vi "phan.vi"() -> ()   [LabVIEW 2019]
uses:
  <vilib>/Platform/TimedLoop/XDataNode/timing_clust.ctl
  <vilib>/Platform/TimedLoop/XDataNode/nitl_modes.ctl
  <vilib>/Platform/TimedLoop/XDataNode/wakeup.ctl
  <vilib>/platform/TimedLoop/XDataNode/XDataNode.xnode
  <vilib>/Platform/TimedLoop/XDataNode/XDNodeRunTimeDep.lvlib
  <vilib>/ptbypt/NI_PtbyPt.lvlib
panel:
  in  "Kdv3":dbl
  in  "Kiv3":dbl=30.0
  in  "Kpv3":dbl=0.6
  in  "Kdv2":dbl
  in  "Kiv2":dbl=30.0
  in  "Kpv2":dbl=0.6
  in  "1000Ts":i64=200
  out "fs":dbl=10.0
  out "TOA DO 2":dbl[][](array[numeric])
  out "sailechS":cluster{"Filtered x":dbl}(graph)
  in  "Kds":dbl
  in  "Kis":dbl
  in  "Kps":dbl=4.0
  in  "?":enum32{"DUONG 2", "DUONGTRON"}(tab)
  in  "S_sp 2":dbl=0.13
  in  "R 2":dbl=0.5
  in  "phi_end 2":dbl=100.0
  in  "R":dbl=0.5
  in  "phi_end":dbl=100.0
  in  "phi_start":dbl=3.14 format="%#_13g"
  in  "step":dbl
  out "V_ph":dbl
  out "V_dk":dbl
  out "w_ph3":dbl
  out "w_ph2":dbl
  out "w_ph1":dbl
  in  "RESETMAP":bool=TRUE caption="Reset"
  out "duty3":dbl
  out "duty2":dbl
  out "duty1":dbl
  in  "RESET":bool
  out "Y_sp":dbl
  out "X_sp":dbl
  out "Y_ph":dbl
  out "X_ph":dbl
  out "Map":cluster{"Y":dbl[], "Y":dbl[]}[](graph)
  out "V3_sp":dbl
  out "V3_ph":dbl
  out "VAN TOC":T1(graph)
  in  "Kdv1":dbl
  in  "Kiv1":dbl=30.0
  in  "Kpv1":dbl=0.6
  out "V2_ph":dbl
  out "V1_ph":dbl
  out "V2_sp":dbl
  out "V1_sp":dbl
  in  "START":bool
  # "HE THONG"
  # "PID VI TRI"
  # "PID TOC DO"
  # "DUTY"
  # "VI TRI DIEU KHIEN\n(m)"
  # "VI TRI PHAN HOI\n(m)"
  # "TOC DO PHAN HOI (rad/s)"
  # "VAN TOC DIEU KHIEN\n(m/s)"
  # "VAN TOC PHAN HOI\n(m/s)"
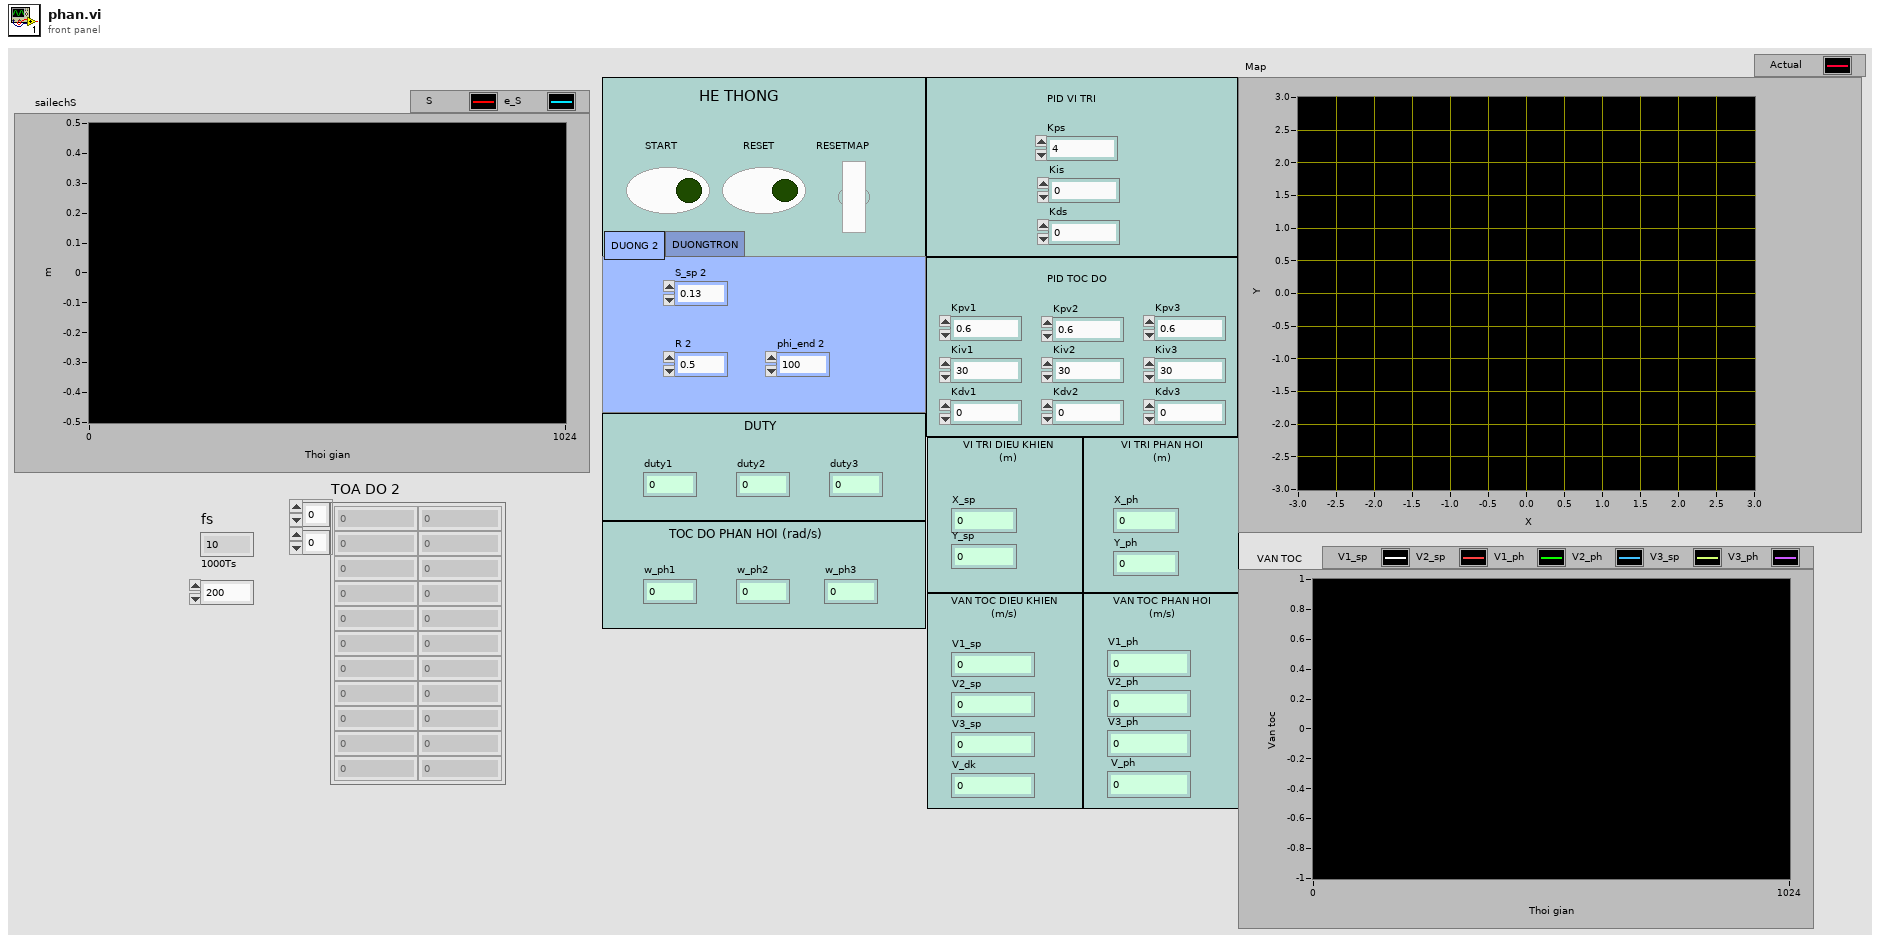
[diagram p1: front panel]
types:
  T1 = cluster{dbl, dbl, "V1_ph":dbl, "V2_ph":dbl, dbl, "V3_ph":dbl}
  T2 = typedef "XDNodeRunTimeDep.lvlib/timing_clust.ctl" = cluster{"Expected End [f-1]":u64, "Actual End [f-1]":u64, "Finished Late? [f-1]":bool, "Expected End [i-1]":u64, "Actual End [i-1]":u64, "Finished Late? [i-1]":bool, "Expected Start [i]":u64, "Actual Start [i]":u64, "Expected Start [f]":u64, "Actual Start [f]":u64, "Source Name":string, "Structure Name":string, "Period":i64, "Deadline":i64, "Offset":i64, "Start":i64, "Priority":i32, "Timeout":i32, "Mode":T3, "Wakeup Reason":T4, "Error":errorcluster, "Source Type":string, "Secondary Source Type":string, "Global End Time":u64, "Global Start Time":u64, "Frame Duration":u64, "Iteration Duration":u64, "Assigned CPU":i32, "I/O Scan Engine Mode":u32}
  T3 = typedef "XDNodeRunTimeDep.lvlib/nitl_modes.ctl" = enum32{"No Change", "Process missed periods, maintain original phase", "Discard missed periods, maintain original phase", "Process missed periods, ignore original phase", "Discard missed periods, ignore original phase"}
  T4 = typedef "XDNodeRunTimeDep.lvlib/wakeup.ctl" = enum32{"Normal", "Aborted", "Asynchronous wakeup", "Timing source error", "Timed loop error", "Timeout"}
  T5 = cluster{"V1_sp":dbl, "V_ph1":dbl, "V2_sp":dbl, "V_ph2":dbl, "V3_sp":dbl, "V_ph3":dbl}
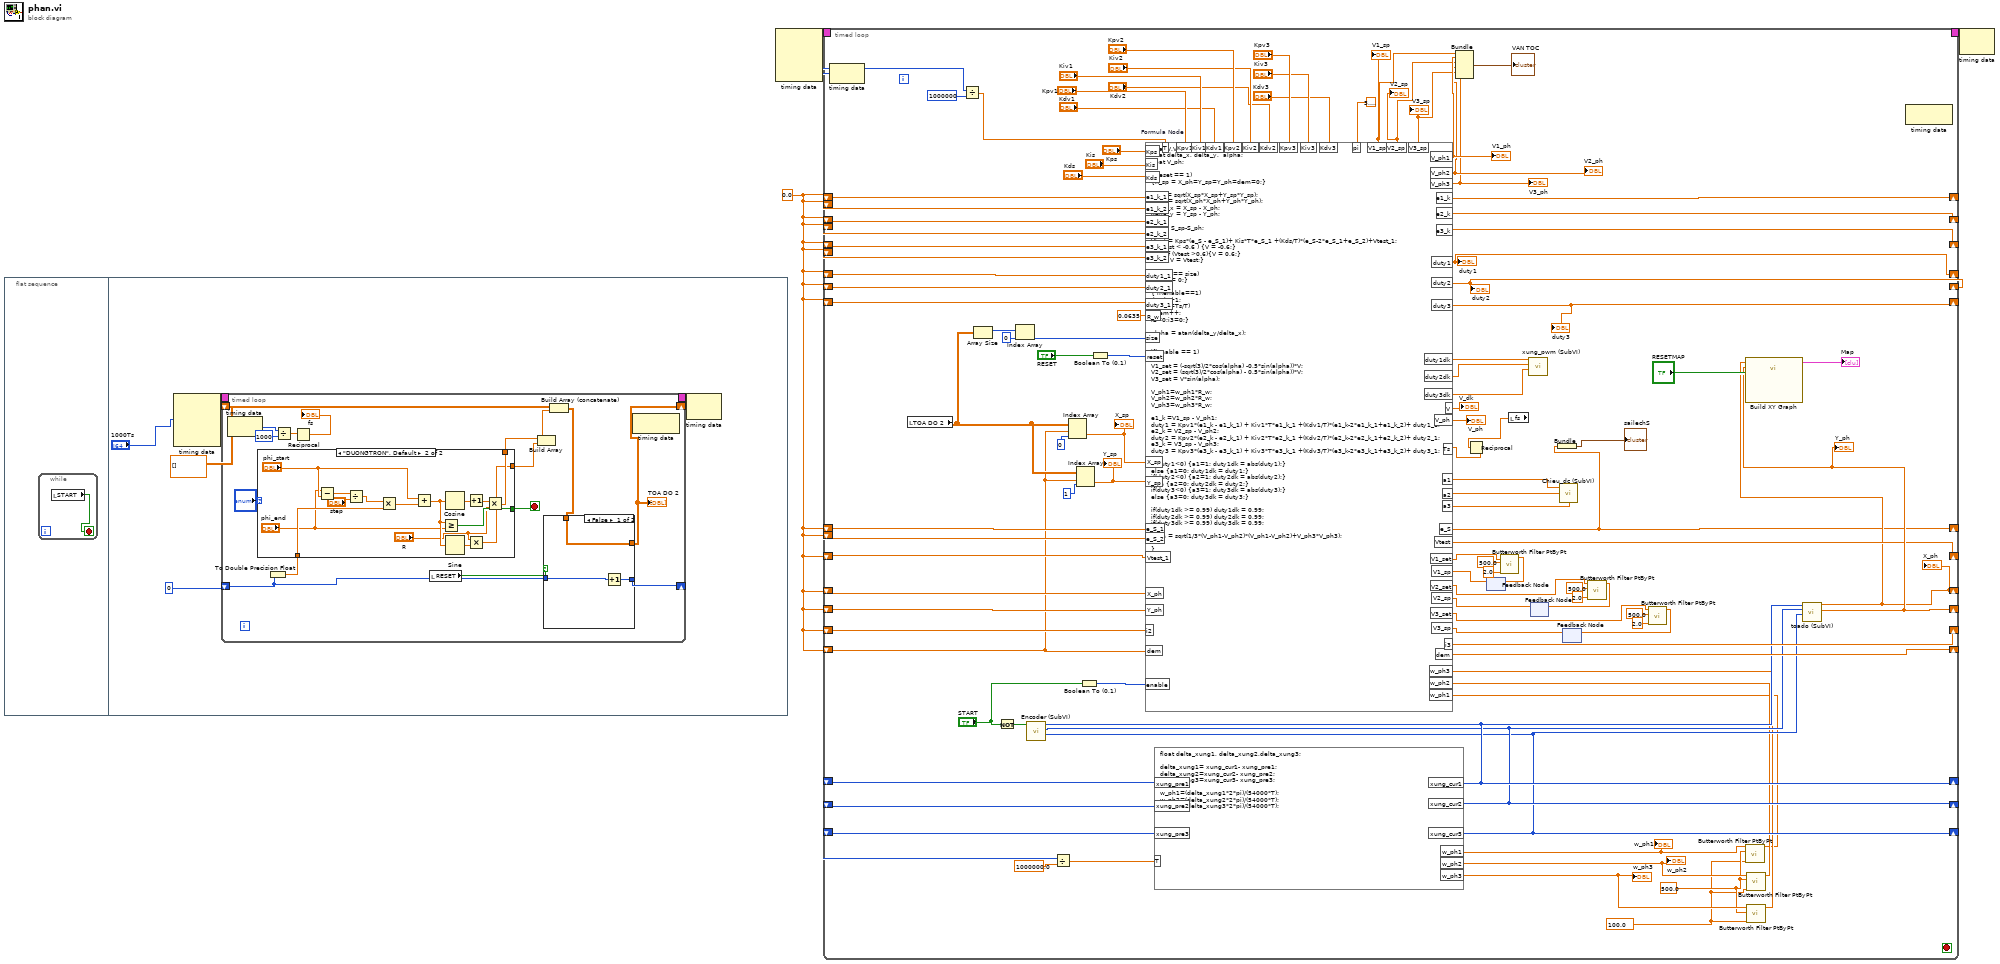
[diagram p0: block diagram]
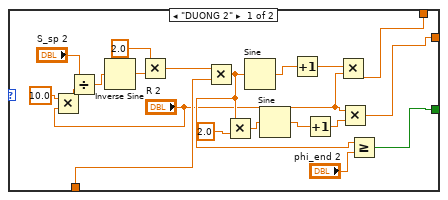
[diagram p2: hidden frame]
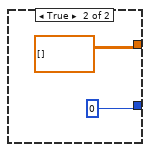
[diagram p3: hidden frame]
diagram:
  w1 = 0.0 ("e1")
  n1 = flat-sequence {
    frame #0 {
      n2 = while {
        stop <- w4 stop-if-true
        n3 = local read "START"() -> (w4:bool)
      }
    }
    frame #1 {
      n4 = node-c288("1000Ts") -> (w9:T2)  [unwired: 3 in]
      n5 = timed-loop {
        timing: w9 -> [_]
        timing-out: [_] -> w8
        shift-right: [w17] -> _
        shift-left: dbl[][] [] -> [w23]
        shift-right: [w21] -> _
        shift-left: 0 -> [w20]
        stop <- w12 stop-if-true
        n6 = node-c288() -> (w16:i64)  [unwired: 1 in]
        n7 = To Double Precision Float(number=w20) -> (double precision float=w25:dbl)
        n8 = case shown="\"DUONGTRON\", Default" "?" {
          tunnel: w25 -> [w45 w60]
          tunnel: [w37 w54] -> w19
          tunnel: [w38 w53] -> w18
          tunnel: [w34 w52] -> w12
          frame "DUONG 2" {
            n9 = Multiply(x=10.0, y="R 2") -> (x*y=w32:dbl)
            n10 = Divide(x="S_sp 2", y=w32) -> (x/y=w29:dbl)
            n11 = Inverse Sine(1:w29) -> (0:w28:dbl)
            n12 = Multiply(x=2.0, y=w28) -> (x*y=w26:dbl)
            n13 = Multiply(x=w26, y=w45) -> (x*y=w35:dbl)
            n14 = Multiply(x=w35, y=2.0) -> (x*y=w40:dbl)
            n15 = Sine(x=w35) -> (sin(x)=w44:dbl)
            n16 = Sine(x=w40) -> (sin(x)=w41:dbl)
            n17 = Increment(x=w44) -> (x+1=w39:dbl)
            n18 = Increment(x=w41) -> (x+1=w42:dbl)
            n19 = Multiply(x=w39, y="R 2") -> (x*y=w37:dbl)
            n20 = Multiply(x="R 2", y=w42) -> (x*y=w38:dbl)
            n21 = Greater Or Equal?(x=w35, y="phi_end 2") -> (x >= y?=w34:bool)
          }
          frame "DUONGTRON", Default {
            n22 = Subtract(x="phi_end", y="phi_start") -> (x-y=w48:dbl)
            n23 = Divide(x=w48, y="step") -> (x/y=w46:dbl)
            n24 = Multiply(x=w46, y=w60) -> (x*y=w59:dbl)
            n25 = Add(x="phi_start", y=w59) -> (x+y=w58:dbl)
            n26 = Greater Or Equal?(x=w58, y="phi_end") -> (x >= y?=w52:bool)
            n27 = Cosine(x=w58) -> (cos(x)=w57:dbl)
            n28 = Sine(x=w58) -> (sin(x)=w55:dbl)
            n29 = Increment(x=w57) -> (x+1=w56:dbl)
            n30 = Multiply(x="R", y=w55) -> (x*y=w53:dbl)
            n31 = Multiply(x=w56, y="R") -> (x*y=w54:dbl)
          }
        }
        n32 = Divide(x=w16, y=i64 1000) -> (x/y=w14:dbl)
        n33 = Reciprocal(x=w14) -> (1/x=→"fs":dbl)
        n34 = local read "RESET"() -> (w11:bool)
        n35 = Build Array(w19, w18) -> (w24:dbl[])
        n36 = Build Array (concatenate)(w23, w24) -> (w22:dbl[][])
        n37 = case shown="False" w11 {
          tunnel: w22 -> [w63 _]
          tunnel: [w63 dbl[][] []] -> w17
          tunnel: [w62 0] -> w21
          tunnel: w20 -> [w61 _]
          frame False {
            n38 = Increment(x=w61) -> (x+1=w62:i32)
          }
          frame True {
          }
        }
        "TOA DO 2" <- w17
        n39 = node-c288() -> ()  [unwired: 1 in, 1 out]
      }
      n40 = node-c288(w8) -> ()  [unwired: 1 out]
    }
  }
  n41 = node-c288() -> (w3:T2)  [unwired: 4 in]
  n42 = timed-loop {
    timing: w3 -> [_]
    timing-out: [_] -> w2
    shift-right: [w181] -> _
    shift-left: w1 -> [w179]
    shift-right: [w180] -> _
    shift-left: w1 -> [w127]
    shift-right: [w172] -> _
    shift-left: w1 -> [w171]
    shift-right: [w91] -> _
    shift-left: w1 -> [w170]
    shift-right: [w149] -> _
    shift-left: w1 -> [w169]
    shift-right: [w168] -> _
    shift-left: w1 -> [w92]
    shift-right: [w147] -> _
    shift-left: w1 -> [w148]
    shift-right: [w146] -> _
    shift-left: w1 -> [w143]
    shift-right: [w145] -> _
    shift-left: w1 -> [w142]
    shift-right: [w144] -> _
    shift-left: w1 -> [w141]
    shift-right: [w130] -> _
    shift-left: _ -> [w138]
    shift-right: [w129] -> _
    shift-left: _ -> [w137]
    shift-right: [w128] -> _
    shift-left: _ -> [w136]
    shift-right: [w74] -> _
    shift-left: w1 -> [w121]
    shift-right: [w119] -> _
    shift-left: w1 -> [w120]
    shift-left: w1 -> [w115]
    shift-left: w1 -> [w114]
    shift-left: w1 -> [w113]
    shift-left: w1 -> [w112]
    stop <- _ stop-if-true
    w106 = 100.0 ("flw")
    w107 = 500.0 ("sampling freq: fs")
    n43 = node-c288() -> (w133:i64)  [unwired: 1 in]
    n44 = local read "TOA DO 2"() -> (w93:dbl[][])
    n45 = Divide(x=w133, y=i64 1000000) -> (x/y=w131:dbl)
    n46 = Array Size(array=w93) -> (size(s)=w164:i32[])
    n47 = Not(x="START") -> (.not. x?=w151:bool)
    n48 = Index Array(array=w164, index=0) -> (element=w162:i32)
    n49 = call "Encoder (SubVI).vi"("Boolean"=w151) -> ("Counter Value3"=w128:i32, "Counter Value 2"=w129:i32, "Counter Value"=w130:i32)  [unwired: 8 in]
    n50 = Divide(x=w133, y=1000000.0) -> (x/y=w134:dbl)
    n51 = Index Array(array=w93, index (row)=w92, index (col)=0 ("disabled index (col)")) -> (element=w166:dbl)
    "X_sp" <- w166
    n52 = Index Array(array=w93, index (row)=w92, index (col)=1 ("disabled index (col)")) -> (element=w165:dbl)
    "Y_sp" <- w165
    n53 = Boolean To (0,1)(Boolean="START") -> (0, 1=w178:i16)
    n54 = Boolean To (0,1)(Boolean="RESET") -> (0, 1=w161:i16)
    n55 = formula code="float delta_xung1, delta_xung2,delta_xung3;\n\ndelta_xung1= xung_cur1- xung_pre1;\ndelta_xung2=xung_cur2- xung_pre2;\ndelta_xung3=xung_cur3- xung_pre3; \n\nw_ph1=(delta_xung1*2*pi)/(54000*T);\nw_ph2=(delta_xung2*2*pi)/(54000*T);\nw_ph3=(delta_xung3*2*pi)/(54000*T);"("xung_pre1"=w138, "xung_pre2"=w137, "xung_pre3"=w136, "xung_cur1"=w130, "xung_cur2"=w129, "xung_cur3"=w128, "T"=w134) -> ("w_ph1"=w95:dbl, "w_ph2"=w109:dbl, "w_ph3"=w108:dbl)
    "w_ph1" <- w95
    "w_ph2" <- w109
    "w_ph3" <- w108
    n56 = feedback #1() -> (w82:dbl)  [unwired: 1 in]
    n57 = local read "fs"() -> (w103:dbl)
    n58 = Reciprocal(x=w103) -> (1/x=w102:dbl)
    n59 = feedback #2() -> (w79:dbl)  [unwired: 1 in]
    n60 = feedback #3() -> (w76:dbl)  [unwired: 1 in]
    n61 = call <vilib>:"Butterworth Filter PtByPt.vi"("low cutoff freq: fl"=w106, "sampling freq: fs"=w107, "x"=w95) -> ("Filtered x"=w94:dbl)  [unwired: 6 in, 1 out]
    n62 = call <vilib>:"Butterworth Filter PtByPt.vi"("low cutoff freq: fl"=w106, "sampling freq: fs"=w107, "x"=w109) -> ("Filtered x"=w105:dbl)  [unwired: 6 in, 1 out]
    n63 = call <vilib>:"Butterworth Filter PtByPt.vi"("low cutoff freq: fl"=w106, "sampling freq: fs"=w107, "x"=w108) -> ("Filtered x"=w104:dbl)  [unwired: 6 in, 1 out]
    n64 = formula code="float V,Vtest, S_sp, S_ph;\nfloat delta_x, delta_y,  alpha;\nfloat V_ph;\n \nif(reset == 1)\n{X_sp = X_ph=Y_sp=Y_ph=dem=0;}\n\nS_sp = sqrt(X_sp*X_sp+Y_sp*Y_sp); \nS_ph = sqrt(X_ph*X_ph+Y_ph*Y_ph); \ndelta_x = X_sp - X_ph;\ndelta_y = Y_sp - Y_ph;\n\ne_S = S_sp-S_ph; \n\nVtest = Kps*(e_S - e_S_1)+ Kis*T*e_S_1 +(Kds/T)*(e_S-2*e_S_1+e_S_2)+Vtest_1;\nif (Vtest < -0.6 ) {V = -0.6;} \nelse if (Vtest >0.6){V = 0.6;}\nelse {V = Vtest;}\n\nif(dem == size)\n{dem = 0;}\nelse\n{ if(enable==1)\n i3=i2+1;\nif (i3>=Ts/T)\n{dem++;\ni2=0;i3=0;}\n\nalpha = atan(delta_y/delta_x);\n\n\nif(enable == 1)\n{\nV1_set = (-sqrt(3)/2*cos(alpha) -0.5*sin(alpha))*V;\nV2_set = (sqrt(3)/2*cos(alpha) - 0.5*sin(alpha))*V;\nV3_set = V*sin(alpha); \n\nV_ph1=w_ph1*R_w;\nV_ph2=w_ph2*R_w;\nV_ph3=w_ph3*R_w;\n\ne1_k =V1_sp - V_ph1;\nduty1 = Kpv1*(e1_k - e1_k_1) + Kiv1*T*e1_k_1 +(Kdv1/T)*(e1_k-2*e1_k_1+e1_k_2)+ duty1_1;\ne2_k = V2_sp - V_ph2;\nduty2 = Kpv2*(e2_k - e2_k_1) + Kiv2*T*e2_k_1 +(Kdv2/T)*(e2_k-2*e2_k_1+e2_k_2)+ duty2_1;\ne3_k = V3_sp - V_ph3;\nduty3 = Kpv3*(e3_k - e3_k_1) + Kiv3*T*e3_k_1 +(Kdv3/T)*(e3_k-2*e3_k_1+e3_k_2)+ duty3_1;\n\nif(duty1<0) {a1=1; duty1dk = abs(duty1);}\nelse {a1=0; duty1dk = duty1;}\nif(duty2<0) {a2=1; duty2dk = abs(duty2);}\nelse {a2=0; duty2dk = duty2;}\nif(duty3<0) {a3=1; duty3dk = abs(duty3);}\nelse {a3=0; duty3dk = duty3;}\n\nif(duty1dk >= 0.99) duty1dk = 0.99;\nif(duty2dk >= 0.99) duty2dk = 0.99;\nif(duty3dk >= 0.99) duty3dk = 0.99;\n\nV_ph = sqrt(1/3*(V_ph1-V_ph2)*(V_ph1-V_ph2)+V_ph3*V_ph3);\n\n}\n}"("Kpv1"="Kpv1", "Kiv1"="Kiv1", "Kdv1"="Kdv1", "pi"=3.141592653589793, "e1_k_1"=w179, "e2_k_1"=w127, "enable"=w178, "T"=w131, "e3_k_1"=w171, "X_ph"=w170, "X_sp"=w166, "Y_sp"=w165, "Y_ph"=w169, "dem"=w92, "size"=w162, "reset"=w161, "i2"=w148, "duty1_1"=w143, "duty2_1"=w142, "duty3_1"=w141, "w_ph1"=w94, "w_ph2"=w105, "w_ph3"=w104, "e_S_1"=w121, "Vtest_1"=w120, "Kps"="Kps", "Kis"="Kis", "Kds"="Kds", "e1_k_2"=w115, "e2_k_2"=w114, "e3_k_2"=w113, "e_S_2"=w112, "Ts"=w102, "Kpv2"="Kpv2", "Kiv2"="Kiv2", "Kdv2"="Kdv2", "Kpv3"="Kpv3", "Kiv3"="Kiv3", "Kdv3"="Kdv3", "V1_sp"=w82, "V2_sp"=w79, "V3_sp"=w76, "R_w"=0.0635 ("input variable")) -> ("V1_sp"=w159:dbl, "V_ph1"=w158:dbl, "V_ph2"=w156:dbl, "e1_k"=w181:dbl, "e2_k"=w180:dbl, "V2_sp"=w157:dbl, "duty1"=w146:dbl, "duty2"=w145:dbl, "e3_k"=w172:dbl, "V_ph3"=w155:dbl, "V3_sp"=w154:dbl, "duty3"=w144:dbl, "a1"=w150:dbl, "a2"=w140:dbl, "a3"=w139:dbl, "dem"=w168:dbl, "i3"=w147:dbl, "duty1dk"=w126:dbl, "duty2dk"=w125:dbl, "duty3dk"=w124:dbl, "V"=→"V_dk":dbl, "V_ph"=→"V_ph":dbl, "e_S"=w74:dbl, "Vtest"=w119:dbl, "V1_set"=w84:dbl, "V2_set"=w81:dbl, "V3_set"=w78:dbl)
    "V1_sp" <- w159
    "V2_sp" <- w157
    "V1_ph" <- w158
    "V2_ph" <- w156
    "V3_ph" <- w155
    "V3_sp" <- w154
    "duty1" <- w146
    "duty2" <- w145
    "duty3" <- w144
    n65 = Bundle("V1_sp"=w159, "V_ph1"=w158, "V2_sp"=w157, "V_ph2"=w156, "V3_sp"=w154, "V_ph3"=w155) -> (→"VAN TOC":T5)  [unwired: 1 in]
    n66 = call <vilib>:"Butterworth Filter PtByPt.vi"("low cutoff freq: fl"=2.0, "sampling freq: fs"=500.0, "x"=w84) -> ("Filtered x"=w83:dbl)  [unwired: 6 in, 1 out]
    n67 = feedback-in #1(w83) -> ()
    n68 = call "xung_pwm (SubVI).vi"("duty3 in"=w124, "duty2 in"=w125, "duty1 in"=w126) -> ()  [unwired: 6 in, 3 out]
    n69 = Bundle("e_S"=w74) -> (→"sailechS":cluster{"e_S":dbl})  [unwired: 1 in]
    n70 = call "Chieu_dc (SubVI).vi"("a3"=w139, "a2"=w140, "a1"=w150) -> ()
    n71 = call <vilib>:"Butterworth Filter PtByPt.vi"("low cutoff freq: fl"=2.0, "sampling freq: fs"=500.0, "x"=w81) -> ("Filtered x"=w80:dbl)  [unwired: 6 in, 1 out]
    n72 = feedback-in #2(w80) -> ()
    n73 = call <vilib>:"Butterworth Filter PtByPt.vi"("low cutoff freq: fl"=2.0, "sampling freq: fs"=500.0, "x"=w78) -> ("Filtered x"=w77:dbl)  [unwired: 6 in, 1 out]
    n74 = feedback-in #3(w77) -> ()
    n75 = call "toado (SubVI).vi"("X3"=w128, "X2"=w129, "X1"=w130) -> ("Y_ph"=w149:dbl, "X_ph"=w91:dbl)  [unwired: 7 in]
    "X_ph" <- w91
    "Y_ph" <- w149
    n76 = call "Build XY Graph"("Reset"="RESETMAP", "Y Input"=w149, "X Input"=w91) -> ("XY Graph"=→"Map":cluster{"X":dbl[], "Y":dbl[]}[])  [unwired: 7 in, 1 out]
    n77 = node-c288() -> ()  [unwired: 1 in, 1 out]
  }
  n78 = node-c288(w2) -> ()  [unwired: 1 out]
